vi "2-3.vi"(6 "kf(Hz/V)":dbl=50000.0, 8 "An(V)":dbl=0.1, 9 "带通Butterworth滤波器":cluster{"中心频率(Hz)":dbl, "带宽(Hz)":dbl}={"中心频率(Hz)"=150000.0, "带宽(Hz)"=280000.0}, 10 "调制信号":cluster{"T(s)":dbl, "Am(V)":dbl}={"T(s)"=0.0002, "Am(V)"=1.0}, 11 "载波信号":cluster{"fc(Hz)":dbl, "Ac(V)":dbl}={"fc(Hz)"=150000.0, "Ac(V)"=1.0}) -> (1 "频域":cluster{"f0":dbl, "df":dbl, "magnitude":dbl[]}(graph), 2 "时域 2":waveform(dbl)[](graph), 3 "时域":waveform(dbl)[](graph))   [LabVIEW 2018]
uses:
  <vilib>/Analysis/3filter.llb/Filter Passband Type.ctl
  <vilib>/Analysis/3filter.llb/Butterworth Filter (DBL).vi
  <vilib>/express/express analysis/Spectral/Block/exnSpectralBlock spectral measurements peak poly.vi
  <vilib>/express/express analysis/Spectral/Block/exnSpectralBlock spectral measurements peak WFM.vi
  <vilib>/express/express analysis/Spectral/XNode/ExpressSpectralMeasurementsBlockNode.xnode
  <vilib>/measure/NI_MABase.lvlib
  <vilib>/Analysis/NI_AALPro.lvlib
  <vilib>/Analysis/NI_AALBase.lvlib
panel:
  out "fh":dbl
  out "fl":dbl
  in  "选项卡控件":enum32{"调制", "滤波", "解调"}(tab)
  out "频域":cluster{"f0":dbl, "df":dbl, "magnitude":dbl[]}(graph)
  out "时域":waveform(dbl)(graph)
  out "BT(Hz)":dbl
  out "数组":dbl[](array[numeric])
  out "调制信号":waveform(dbl)(graph)
  out "积分信号":waveform(dbl)(graph)
  out "采样参数（采样频率fs，采样数Ns）":cluster{dbl, dbl} {"?" format="%#_6f"; "?" format="%#_6f"}
  out "载波信号":waveform(dbl)(graph)
  # "要显示n个周期的调制信号波形，\n则采样数Ns=n*fs/fm"
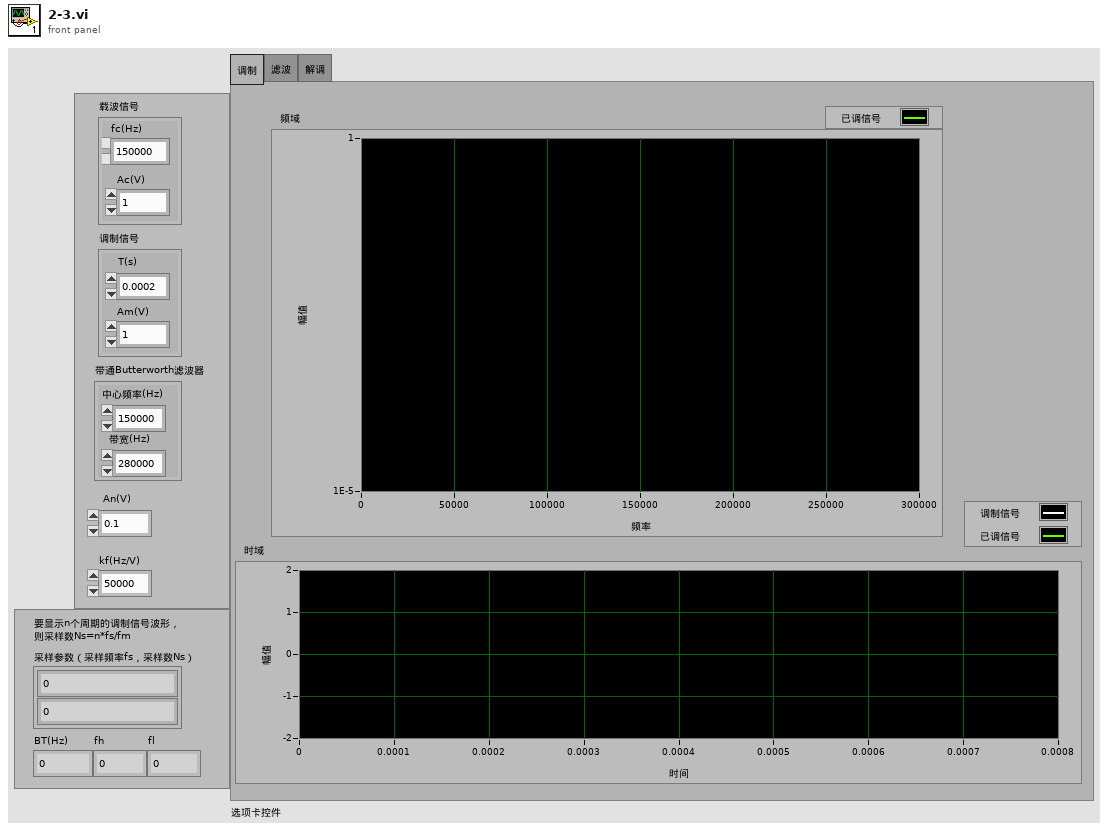
[diagram p1: front panel]
types:
  T1 = typedef "NI_AALBase.lvlib/Filter Passband Type.ctl" = enum32{"Lowpass", "Highpass", "Bandpass", "Bandstop"}
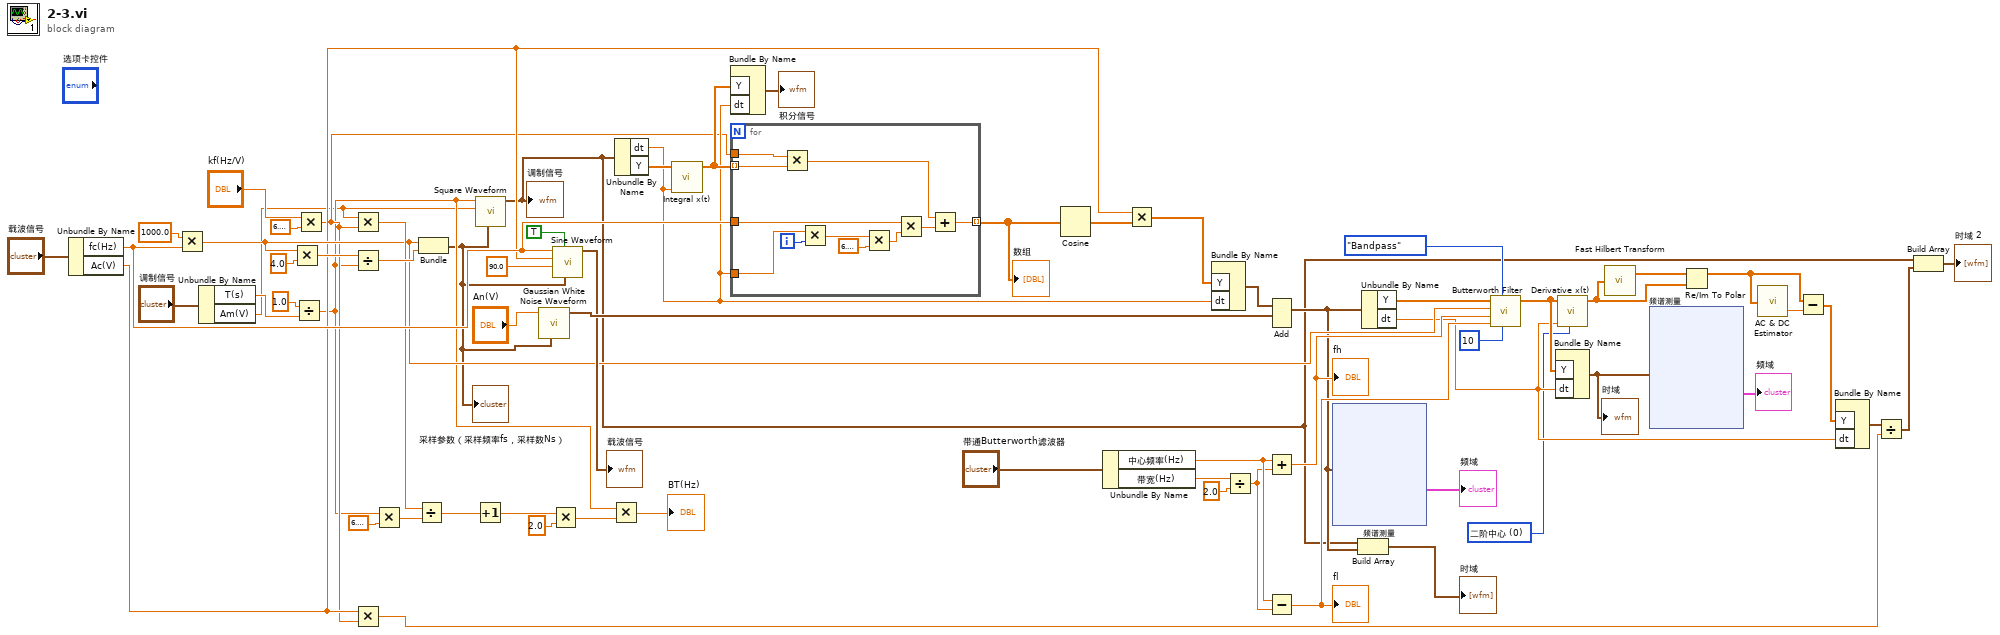
[diagram p0: block diagram]
diagram:
  w19 = u16 0 items=["二阶中心", "四阶中心", "前向", "后向"] ("method")
  n1 = Unbundle By Name("载波信号") -> ("fc(Hz)"=w55:dbl, "Ac(V)"=w15:dbl)
  n2 = Multiply(x=1000.0, y=w55) -> (x*y=w27:dbl)
  n3 = Unbundle By Name("调制信号") -> ("T(s)"=w5:dbl, "Am(V)"=w3:dbl)
  n4 = Multiply(x=w27, y=4.0) -> (x*y=w61:dbl)
  n5 = Divide(x=1.0, y=w5) -> (x/y=w4:dbl)
  n6 = Multiply(x="kf(Hz/V)", y=6.283185307179586) -> (x*y=w9:dbl)
  n7 = Multiply(x=w3, y=w9) -> (x*y=w42:dbl)
  n8 = Divide(x=w61, y=w4) -> (x/y=w60:dbl)
  n9 = Multiply(x=w15, y=w9) -> (x*y=w13:dbl)
  n10 = Multiply(x=w4, y=6.283185307179586) -> (x*y=w43:dbl)
  n11 = Divide(x=w42, y=w43) -> (x/y=w41:dbl)
  n12 = Bundle(w27, w60) -> (w2:cluster{dbl, dbl})  [unwired: 1 in]
  "采样参数（采样频率fs，采样数Ns）" <- w2
  n13 = Increment(x=w41) -> (x+1=w40:dbl)
  n14 = call <vilib>:"Square Waveform.vi"("sampling info"=w2, "amplitude"=w3, "frequency"=w4) -> ("signal out"=w1:waveform(dbl))  [unwired: 7 in, 1 out]
  "调制信号" <- w1
  n15 = call <vilib>:"Gaussian White Noise Waveform.vi"("sampling info"=w2, "standard deviation"="An(V)") -> ("signal out"=w47:waveform(dbl))  [unwired: 8 in, 1 out]
  n16 = Multiply(x=w40, y=2.0) -> (x*y=w38:dbl)
  n17 = call <vilib>:"Sine Waveform.vi"("sampling info"=w2, "reset signal"=TRUE, "phase"=90.0, "amplitude"=w15, "frequency"=w55) -> ("signal out"=→"载波信号":waveform(dbl))  [unwired: 5 in, 1 out]
  n18 = Multiply(x=w4, y=w38) -> (x*y=→"BT(Hz)":dbl)
  n19 = Unbundle By Name(w1) -> ("dt"=w52:dbl, "Y"=w62:dbl[])
  n20 = call <vilib>:"Integral x(t).vi"("dt"=w52, "X"=w62) -> ("Integral X"=w56:dbl[])  [unwired: 8 in, 1 out]
  n21 = Bundle By Name("Y"=w56, "dt"=w52) -> (→"积分信号":waveform(dbl))  [unwired: 1 in]
  n22 = for {
    tunnel: w56 -> [w77] mode=indexing
    tunnel: w52 -> [w75]
    tunnel: w55 -> [w71]
    tunnel: [w68] -> w54 mode=indexing
    tunnel: w9 -> [w67]
    i -> [w76]
    n23 = Multiply(x=w67, y=w77) -> (x*y=w69:dbl)
    n24 = Multiply(x=w75, y=w76) -> (x*y=w73:dbl)
    n25 = Multiply(x=w73, y=6.283185307179586) -> (x*y=w72:dbl)
    n26 = Multiply(x=w71, y=w72) -> (x*y=w70:dbl)
    n27 = Add(x=w69, y=w70) -> (x+y=w68:dbl)
  }
  "数组" <- w54
  n28 = Cosine(x=w54) -> (cos(x)=w53:dbl[])
  n29 = Unbundle By Name("带通Butterworth滤波器") -> ("中心频率(Hz)"=w29:dbl, "带宽(Hz)"=w33:dbl)
  n30 = Multiply(x=w15, y=w53) -> (x*y=w51:dbl[])
  n31 = Bundle By Name("Y"=w51, "dt"=w52) -> (w49:waveform(dbl))  [unwired: 1 in]
  n32 = Divide(x=w33, y=2.0) -> (x/y=w28:dbl)
  n33 = Add(1:w47, 2:w49) -> (0:w25:waveform(dbl))  [unwired: 1 in, 1 out]
  n34 = Add(x=w29, y=w28) -> (x+y=w31:dbl)
  "fh" <- w31
  n35 = Subtract(x=w29, y=w28) -> (x-y=w30:dbl)
  "fl" <- w30
  n36 = xnode "频谱测量"("信号"=w25) -> ("FFT - （峰值）"=→"频域":cluster{"f0":dbl, "df":dbl, "magnitude":dbl[]})  [unwired: 1 in, 2 out]
  n37 = Build Array(w1, w25) -> (→"时域":waveform(dbl)[])
  n38 = Unbundle By Name(w25) -> ("Y"=w24:dbl[], "dt"=w20:dbl)
  n39 = call-poly <vilib>:"Butterworth Filter.vi"("order"=10, "filter type"=Filter_Passband_Type."Bandpass", "low cutoff freq: fl"=w30, "high cutoff freq: fh"=w31, "sampling freq: fs"=w27, "X"=w24) -> ("Filtered X"=w22:dbl[])  [unwired: 2 in, 1 out]
  n40 = Bundle By Name("Y"=w22, "dt"=w20) -> (w23:waveform(dbl))  [unwired: 1 in]
  "时域" <- w23
  n41 = call <vilib>:"Derivative x(t).vi"("method"=w19, "dt"=w20, "X"=w22) -> ("dX/dt"=w12:dbl[])  [unwired: 7 in, 1 out]
  n42 = call <vilib>:"Fast Hilbert Transform.vi"("X"=w12) -> ("Hilbert{X}"=w21:dbl[])  [unwired: 1 out]
  n43 = xnode "频谱测量"("信号"=w23) -> ("FFT - （峰值）"=→"频域":cluster{"f0":dbl, "df":dbl, "magnitude":dbl[]})  [unwired: 1 in, 2 out]
  n44 = Re/Im To Polar(2:w12, 3:w21) -> (1:w18:dbl[])  [unwired: 1 out]
  n45 = call <vilib>:"AC & DC Estimator.vi"("Signal (V)"=w18) -> ("DC estimate (V)"=w17:dbl)  [unwired: 1 out]
  n46 = Subtract(x=w18, y=w17) -> (x-y=w16:dbl[])
  n47 = Bundle By Name("Y"=w16, "dt"=w20) -> (w14:waveform(dbl))  [unwired: 1 in]
  n48 = Divide(x=w14, y=w13) -> (x/y=w8:waveform(dbl))
  n49 = Build Array(w1, w8) -> (→"时域 2":waveform(dbl)[])
